vi "local.vi"() -> ()   [LabVIEW 2018]
panel:
  in  "정지":bool
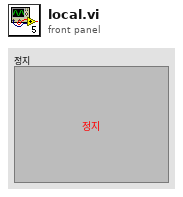
[diagram p1: front panel]
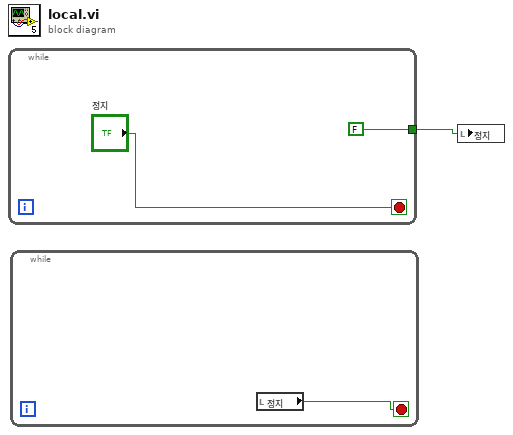
[diagram p0: block diagram]
diagram:
  n1 = while {
    tunnel: [FALSE] -> w1
    stop <- "정지" stop-if-true
  }
  n2 = while {
    stop <- w4 stop-if-true
    n3 = local read "정지"() -> (w4:bool)
  }
  n4 = local write "정지"(w1) -> ()
